vi "1.1 Output Limit.vi"(1 "Direct Voltage":fxp<+/-,20,5>) -> (0 "Steering Limited":fxp<+/-,20,5>)   [LabVIEW 2011]
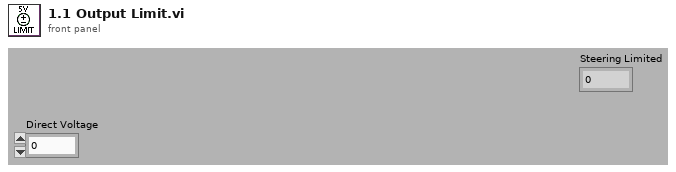
[diagram p1: front panel]
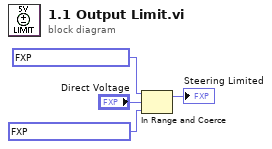
[diagram p0: block diagram]
diagram:
  n1 = In Range and Coerce(upper limit=fxp<+/-,20,5> 5.0 ("y"), x="Direct Voltage", lower limit=fxp<+/-,20,5> -5.0 ("y")) -> (coerced(x)=→"Steering Limited":fxp<+/-,20,5>)  [unwired: 1 out]
